vi "CreateLogFilePath.vi"(8 "error in (no error)":errorcluster) -> (0 "error out":errorcluster, 3 "LoggerPath":path)   [LabVIEW 2021, in "Event Logger.lvlib"]
uses:
  Event Logger.lvlib
  <vilib>/Utility/sysdir.llb/System Directory Type.ctl
  Converter/Path Functions/Path Functions.lvlib
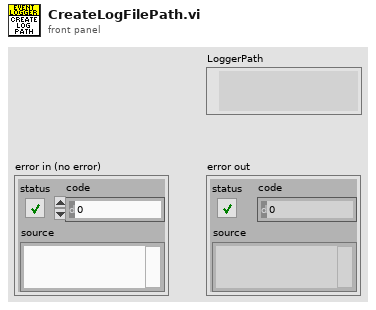
[diagram p1: front panel]
types:
  T1 = typedef "System Directory Type.ctl" = i32
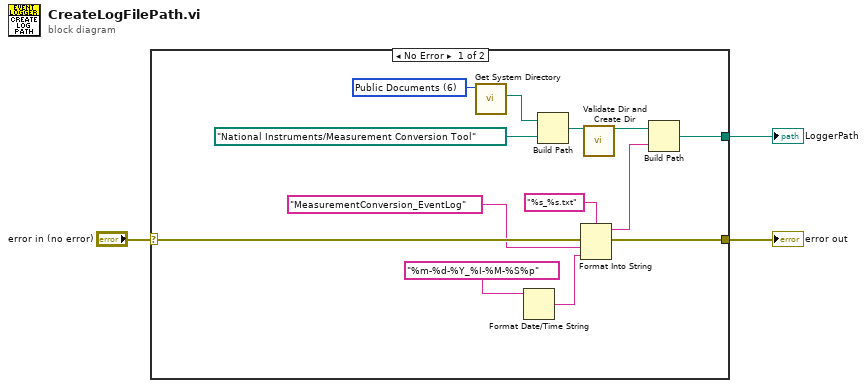
[diagram p0: block diagram]
diagram:
  n1 = case shown="No Error" "error in (no error)" {
    selector: "error in (no error)" -> [w16 w17]
    tunnel: [w10 _] -> w2
    tunnel: [w8 w17] -> w1
    frame No Error {
      w11 = T1 6 items=["User Home"=0, "User Desktop"=1, "User Documents"=2, "User Application Data"=3, "User Preferences"=4, "User Temporary"=5, "Public Documents"=6, "Public Application Data"=7, "Public Preferences"=8, "Public Cache"=13, "System Core Libraries"=9, "System Installed Libraries"=10, "Application Files"=11, "Boot Volume Root"=12] ("system directory type")
      n2 = call <vilib>:"Get System Directory.vi"("system directory type"=w11) -> ("system directory"=w14:path)  [unwired: 10 in]
      n3 = Format Date/Time String(time format string (%c)="%m-%d-%Y_%I-%M-%S%p") -> (date/time string=w5:string)  [unwired: 2 in]
      n4 = Build Path(base path=w14, name or relative path=path "National Instruments/Measurement Conversion Tool" ("Application Directory")) -> (appended path=w15:path)
      n5 = Format Into String(format string="%s_%s.txt", error in=w16, "MeasurementConversion_EventLog" ("name"), w5) -> (resulting string=w9:string, error out=w8:errorcluster)  [unwired: 1 in]
      n6 = call "Validate Dir and Create Dir.vi"("Directory"=w15) -> ("Dup Directory"=w12:path)  [unwired: 13 in, 1 out]
      n7 = Build Path(base path=w12, name or relative path=w9) -> (appended path=w10:path)
    }
    frame Error {
    }
  }
  "LoggerPath" <- w2
  "error out" <- w1
